vi "dfd_Roots Zero-INF Remover.vi"(11 "roots":cdb[](array[numeric])) -> (2 "# zero root":i32, 3 "new roots":cdb[](array[numeric]))   [LabVIEW 2017, in "NI_DigFilterLicensed.lvlib"]
uses:
  <vilib>/addons/Digital Filter Design/NI_DigFilterLicensed.lvlib
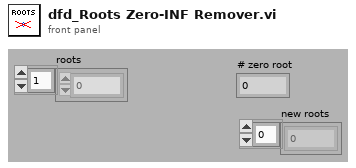
[diagram p1: front panel]
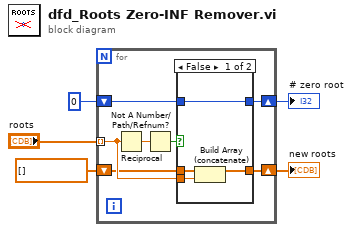
[diagram p0: block diagram]
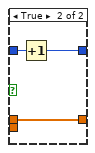
[diagram p2: hidden frame]
diagram:
  n1 = for {
    tunnel: "roots" -> [w7] mode=indexing
    shift-right: [w10] -> w1
    shift-left: 0 -> [w9]
    shift-right: [w8] -> w2
    shift-left: cdb[] [] -> [w6]
    n2 = Reciprocal(x=w7) -> (1/x=w12:cdb)
    n3 = Not A Number/Path/Refnum?(number/path/refnum=w12) -> (NaN/Path/Refnum?=w11:bool)
    n4 = case shown="False" w11 {
      tunnel: [w16 w19] -> w10
      tunnel: w9 -> [w16 w18]
      tunnel: [w15 w17] -> w8
      tunnel: w7 -> [w14 _]
      tunnel: w6 -> [w13 w17]
      frame False {
        n5 = Build Array (concatenate)(w13, w14) -> (w15:cdb[])
      }
      frame True {
        n6 = Increment(x=w18) -> (x+1=w19:i32)
      }
    }
  }
  "new roots" <- w2
  "# zero root" <- w1
